vi "podControl_9066.vi"() -> ()   [LabVIEW 2016]
uses:
  <vilib>/platform/TimedLoop/XDataNode/XDataNode.xnode
  <vilib>/Platform/TimedLoop/XDataNode/nitl_modes.ctl
  <vilib>/Platform/TimedLoop/XDataNode/XDNodeRunTimeDep.lvlib
  <vilib>/Platform/TimedLoop/XDataNode/wakeup.ctl
  <vilib>/Platform/TimedLoop/XDataNode/timing_clust.ctl
  podGlobals_9066.vi
  <vilib>/Platform/TimedLoop/XDataNode/loadnilvce.vi
panel:
  out "Fatality":bool
  in  "Kill":bool
  out "Velocity":bool
  out "Acceleration":bool
  out "Battery Voltage":bool
  out "Internal Pressure":bool
  out "Internal Temperature":bool
  out "Battery Pressure":bool
  out "Battery Temperature":bool
  in  "Latch":bool
  out "Coast Time (s)":dbl
  out "Start Time (s)":dbl
  out "On Time (s)":dbl
  out "FR:":dbl
  out "BL:":dbl
  out "FL:":dbl
  out "BR:":dbl
  in  "Coast (s)":dbl
  in  "RESET":bool
  in  "Velocity (m/s)":dbl
  in  "Timeout (s)":dbl
  out "Internal Pressure (atm)":dbl(slide) scale=0.0..2.0
  out "Internal Temperature (F)":dbl(slide) scale=50.0..120.0
  out "READY":bool
  out "Flight Time (s)":dbl
  in  "START":bool
  out "Acceleration (m/s^2)":dbl(knob) scale=-30.0..30.0
  out "Position (m)":dbl
  out "Velocity (m/s)":dbl(knob) scale=0.0..300.0
  out "Latched":bool
  out "Pusher Engaged":bool
  out "Front Brake Engaged":bool
  out "Back Brake Engaged":bool
  in  "Flight Profile":T1(radio)
  out "Progress":u8(slide) caption="Profile Progress" scale=0.0..100.0
  out "Battery Pressure (atm)":dbl(slide) scale=0.0..2.0
  out "Battery Temperature (F)":dbl(slide) scale=50.0..120.0
  in  "STOP":bool
  out "Battery Voltage":dbl(knob) scale=22.0..26.0
  # "Z-Height (mm)"
  # "Custom:"
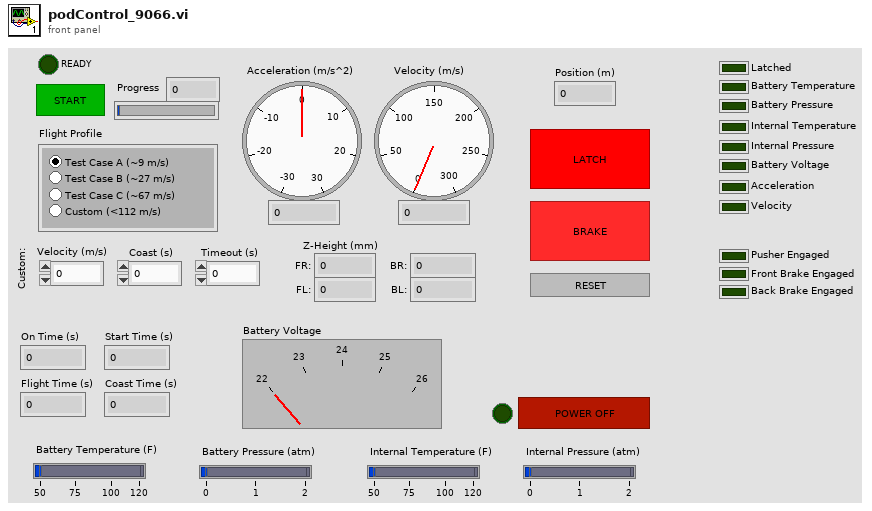
[diagram p1: front panel]
types:
  T1 = enum32{"Test Case A (~9 m/s)", "Test Case B (~27 m/s)", "Test Case C (~67 m/s)", "Custom (<112 m/s)"}
  T2 = typedef "XDNodeRunTimeDep.lvlib/timing_clust.ctl" = cluster{"Expected End [f-1]":u64, "Actual End [f-1]":u64, "Finished Late? [f-1]":bool, "Expected End [i-1]":u64, "Actual End [i-1]":u64, "Finished Late? [i-1]":bool, "Expected Start [i]":u64, "Actual Start [i]":u64, "Expected Start [f]":u64, "Actual Start [f]":u64, "Source Name":string, "Structure Name":string, "Period":i64, "Deadline":i64, "Offset":i64, "Start":i64, "Priority":i32, "Timeout":i32, "Mode":T3, "Wakeup Reason":T4, "Error":errorcluster, "Source Type":string, "Secondary Source Type":string, "Global End Time":u64, "Global Start Time":u64, "Frame Duration":u64, "Iteration Duration":u64, "Assigned CPU":i32, "I/O Scan Engine Mode":u32}
  T3 = typedef "XDNodeRunTimeDep.lvlib/nitl_modes.ctl" = enum32{"No Change", "Process missed periods, maintain original phase", "Discard missed periods, maintain original phase", "Process missed periods, ignore original phase", "Discard missed periods, ignore original phase"}
  T4 = typedef "XDNodeRunTimeDep.lvlib/wakeup.ctl" = enum32{"Normal", "Aborted", "Asynchronous wakeup", "Timing source error", "Timed loop error", "Timeout"}
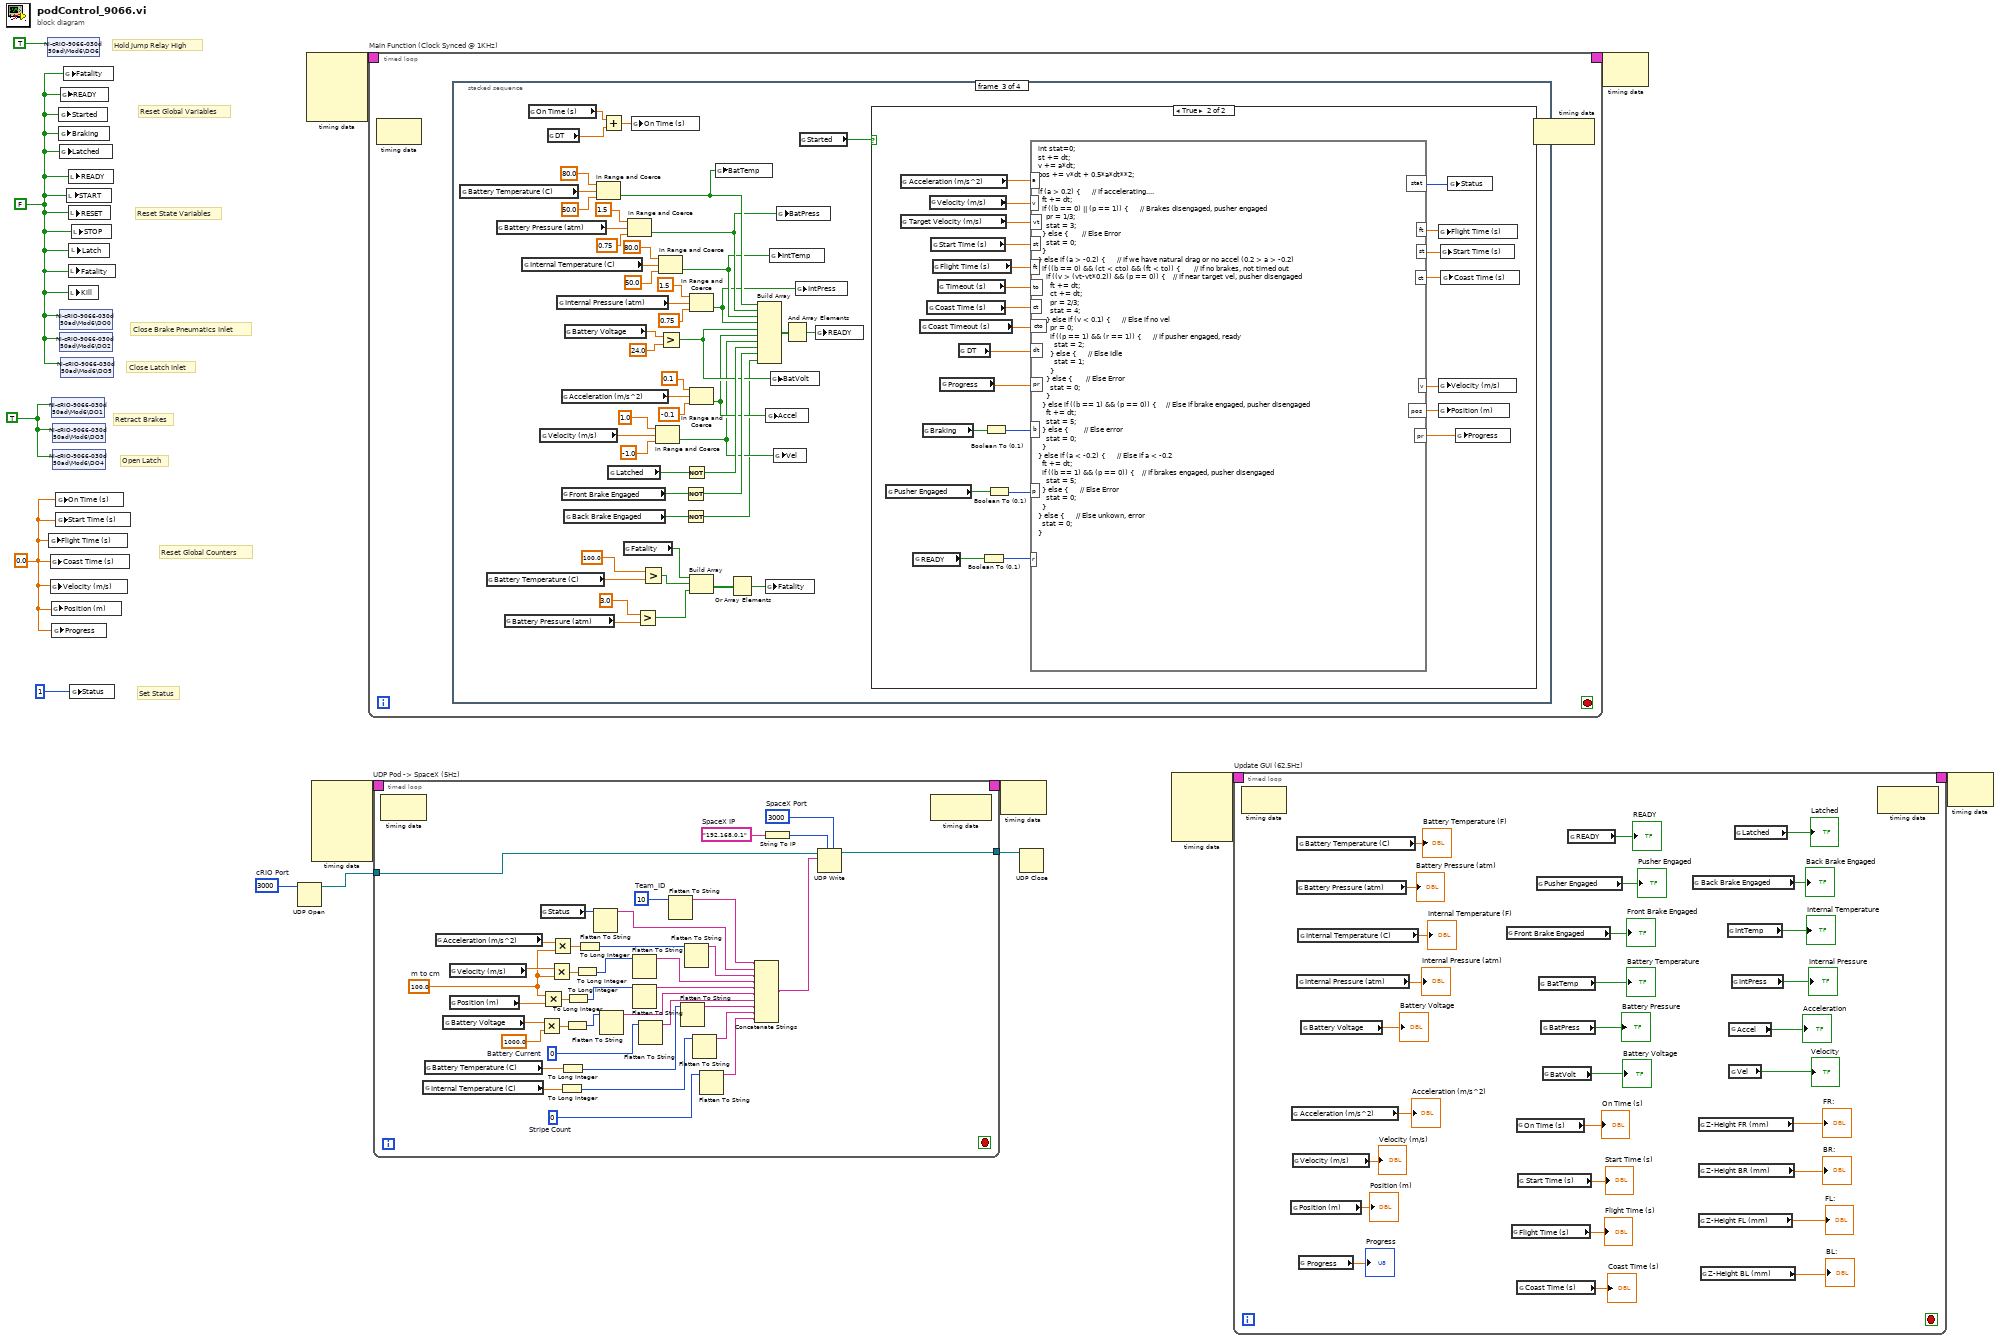
[diagram p0: block diagram]
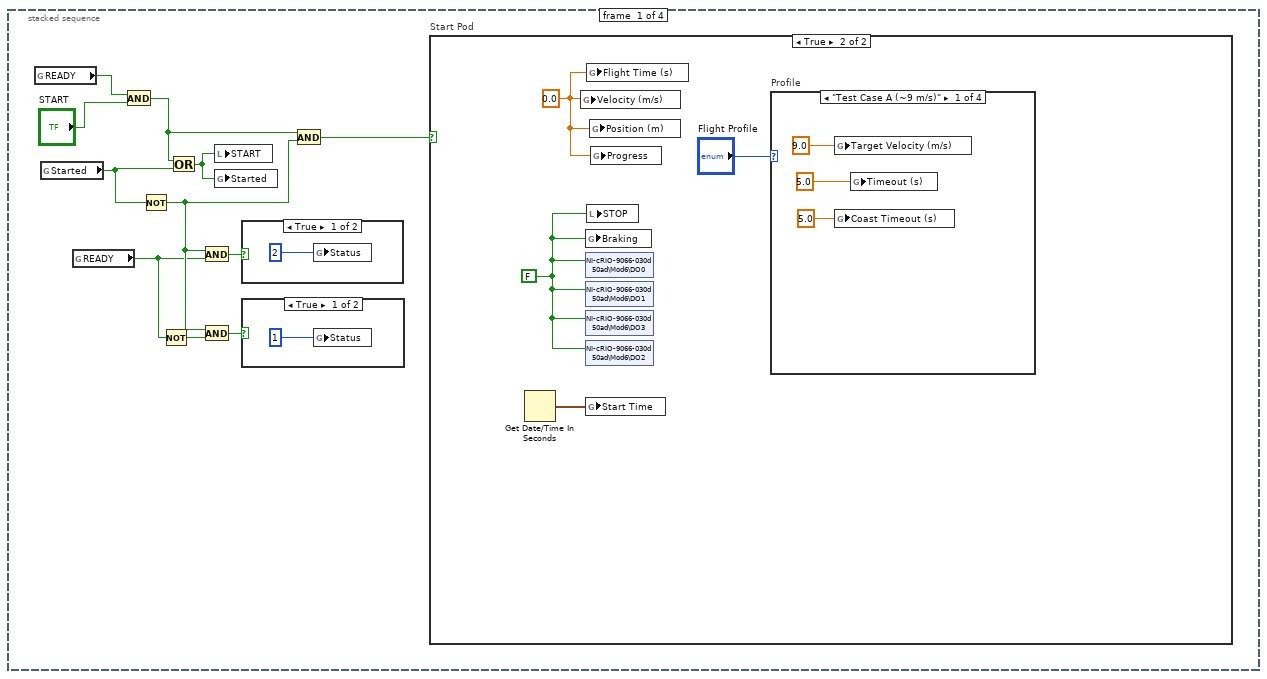
[diagram p2: hidden frame]
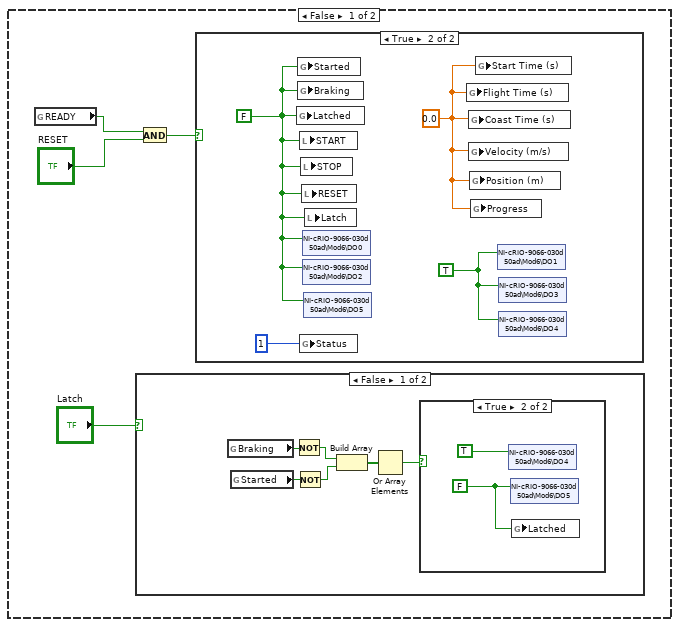
[diagram p5: hidden frame]
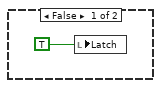
[diagram p6: hidden frame]
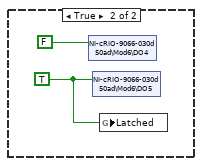
[diagram p7: hidden frame]
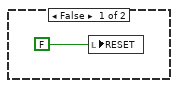
[diagram p8: hidden frame]
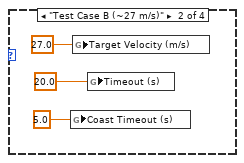
[diagram p9: hidden frame]
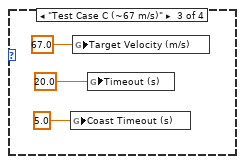
[diagram p10: hidden frame]
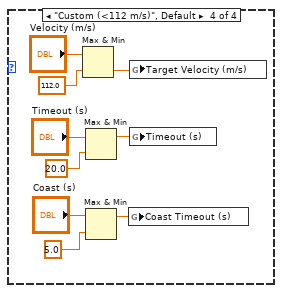
[diagram p11: hidden frame]
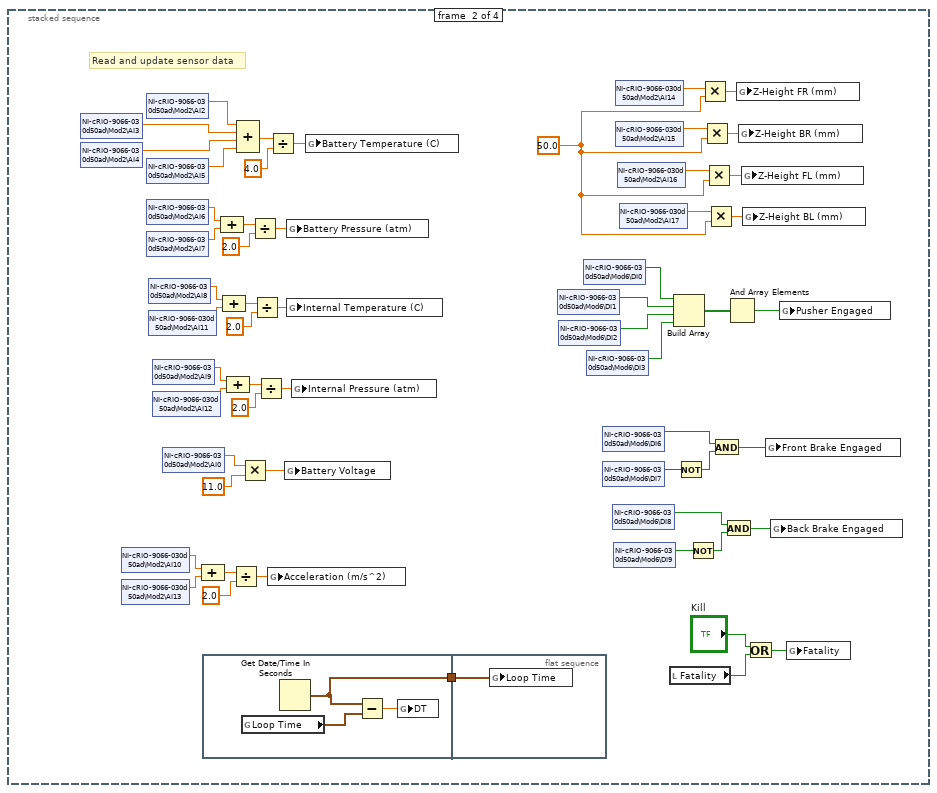
[diagram p12: hidden frame]
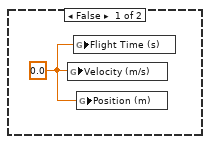
[diagram p13: hidden frame]
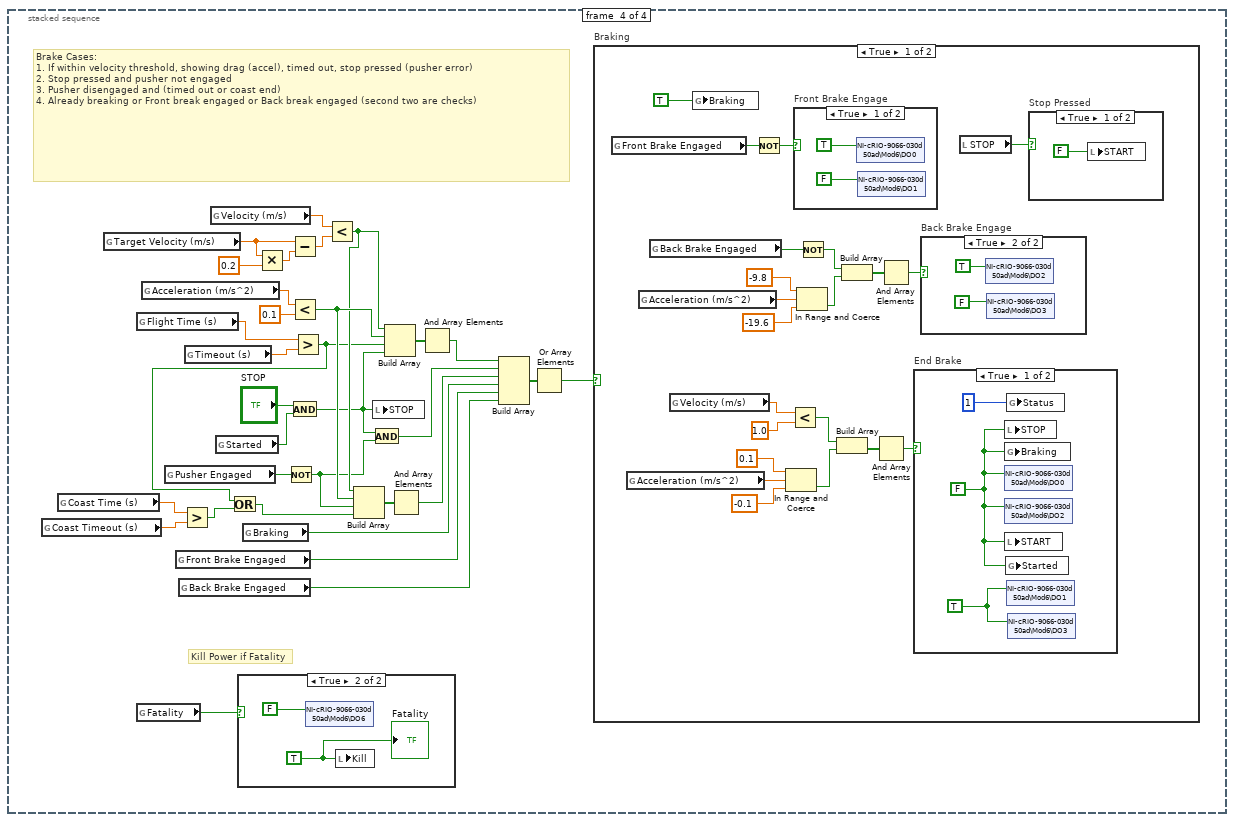
[diagram p14: hidden frame]
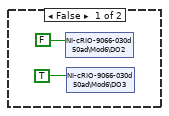
[diagram p16: hidden frame]
diagram:
  w3 = TRUE
  w10 = u32 3000  # cRIO Port
  w1 = FALSE
  w8 = 0.0
  # "Hold Jump Relay High"
  # "Close Latch Inlet"
  # "Open Latch"
  # "Set Status"
  # "Reset Global Counters"
  # "Reset Global Variables"
  # "Reset State Variables"
  # "Close Brake Pneumatics Inlet"
  # "Retract Brakes"
  n1 = shared-variable "NI-cRIO-9066-030d50ad\\Mod6\\DO6"(TRUE) -> ()  [unwired: 1 in, 1 out]
  n2 = global write "podGlobals_9066.vi" "Flight Time (s)"(w8) -> ()
  n3 = global write "podGlobals_9066.vi" "Coast Time (s)"(w8) -> ()
  n4 = global write "podGlobals_9066.vi" "Velocity (m/s)"(w8) -> ()
  n5 = global write "podGlobals_9066.vi" "Position (m)"(w8) -> ()
  n6 = shared-variable "NI-cRIO-9066-030d50ad\\Mod6\\DO1"(w3) -> ()  [unwired: 1 in, 1 out]
  n7 = global write "podGlobals_9066.vi" "Progress"(w8) -> ()
  n8 = shared-variable "NI-cRIO-9066-030d50ad\\Mod6\\DO3"(w3) -> ()  [unwired: 1 in, 1 out]
  n9 = shared-variable "NI-cRIO-9066-030d50ad\\Mod6\\DO4"(w3) -> ()  [unwired: 1 in, 1 out]
  n10 = global write "podGlobals_9066.vi" "On Time (s)"(w8) -> ()
  n11 = global write "podGlobals_9066.vi" "Start Time (s)"(w8) -> ()
  n12 = global write "podGlobals_9066.vi" "Started"(w1) -> ()
  n13 = global write "podGlobals_9066.vi" "Braking"(w1) -> ()
  n14 = global write "podGlobals_9066.vi" "Latched"(w1) -> ()
  n15 = shared-variable "NI-cRIO-9066-030d50ad\\Mod6\\DO0"(w1) -> ()  [unwired: 1 in, 1 out]
  n16 = shared-variable "NI-cRIO-9066-030d50ad\\Mod6\\DO2"(w1) -> ()  [unwired: 1 in, 1 out]
  n17 = global write "podGlobals_9066.vi" "READY"(w1) -> ()
  n18 = shared-variable "NI-cRIO-9066-030d50ad\\Mod6\\DO5"(w1) -> ()  [unwired: 1 in, 1 out]
  n19 = global write "podGlobals_9066.vi" "Fatality"(w1) -> ()
  n20 = local write "START"(w1) -> ()
  n21 = local write "READY"(w1) -> ()
  n22 = local write "RESET"(w1) -> ()
  n23 = local write "Fatality"(w1) -> ()
  n24 = local write "Kill"(w1) -> ()
  n25 = local write "Latch"(w1) -> ()
  n26 = global write "podGlobals_9066.vi" "Status"(1) -> ()
  n27 = local write "STOP"(w1) -> ()
  n28 = UDP Open(11:w10) -> (port=w5:refnum<k16>)  [unwired: 4 in, 2 out]
  n29 = node-c288() -> (w14:T2)  [unwired: 4 in]
  n30 = node-c288() -> (w12:T2)  [unwired: 5 in]
  n31 = timed-loop "Main Function (Clock Synced @ 1KHz)" {
    timing: w14 -> [_]
    timing-out: [_] -> w13
    stop <- _ stop-if-true
    n32 = node-c288() -> ()  [unwired: 1 in, 1 out]
    n33 = stacked-sequence {
      frame #0 {
        n34 = global read "podGlobals_9066.vi" "READY"() -> (w24:bool)
        n35 = global read "podGlobals_9066.vi" "Started"() -> (w25:bool)
        n36 = global read "podGlobals_9066.vi" "READY"() -> (w15:bool)
        n37 = And(x=w24, y="START") -> (x .and. y?=w21:bool)
        n38 = Not(x=w25) -> (.not. x?=w17:bool)
        n39 = Not(x=w15) -> (.not. x?=w16:bool)
        n40 = Or(x=w21, y=w25) -> (x .or. y?=w20:bool)
        n41 = And(x=w17, y=w15) -> (x .and. y?=w19:bool)
        n42 = And(x=w17, y=w16) -> (x .and. y?=w18:bool)
        n43 = local write "START"(w20) -> ()
        n44 = global write "podGlobals_9066.vi" "Started"(w20) -> ()
        n45 = case shown="True" w19 {
          frame True {
            n46 = global write "podGlobals_9066.vi" "Status"(2) -> ()
          }
          frame False {
          }
        }
        n47 = case shown="True" w18 {
          frame True {
            n48 = global write "podGlobals_9066.vi" "Status"(1) -> ()
          }
          frame False {
          }
        }
        n49 = And(x=w21, y=w17) -> (x .and. y?=w22:bool)
        n50 = case "Start Pod" shown="True" w22 {
          frame False {
            n51 = global read "podGlobals_9066.vi" "READY"() -> (w30:bool)
            n52 = case shown="False" "Latch" {
              frame False {
                n53 = global read "podGlobals_9066.vi" "Braking"() -> (w37:bool)
                n54 = global read "podGlobals_9066.vi" "Started"() -> (w36:bool)
                n55 = Not(x=w37) -> (.not. x?=w34:bool)
                n56 = Not(x=w36) -> (.not. x?=w35:bool)
                n57 = Build Array(w34, w35) -> (w33:bool[])
                n58 = Or Array Elements(Boolean array=w33) -> (logical OR=w32:bool)
                n59 = case shown="True" w32 {
                  frame False {
                    n60 = local write "Latch"(TRUE) -> ()
                  }
                  frame True {
                    w39 = FALSE
                    n61 = shared-variable "NI-cRIO-9066-030d50ad\\Mod6\\DO4"(TRUE) -> ()  [unwired: 1 in, 1 out]
                    n62 = shared-variable "NI-cRIO-9066-030d50ad\\Mod6\\DO5"(w39) -> ()  [unwired: 1 in, 1 out]
                    n63 = global write "podGlobals_9066.vi" "Latched"(w39) -> ()
                  }
                }
              }
              frame True {
                w41 = TRUE
                n64 = shared-variable "NI-cRIO-9066-030d50ad\\Mod6\\DO4"(FALSE) -> ()  [unwired: 1 in, 1 out]
                n65 = shared-variable "NI-cRIO-9066-030d50ad\\Mod6\\DO5"(w41) -> ()  [unwired: 1 in, 1 out]
                n66 = global write "podGlobals_9066.vi" "Latched"(w41) -> ()
              }
            }
            n67 = And(x=w30, y="RESET") -> (x .and. y?=w29:bool)
            n68 = case shown="True" w29 {
              frame False {
                n69 = local write "RESET"(FALSE) -> ()
              }
              frame True {
                w45 = TRUE
                w46 = 0.0
                w44 = FALSE
                n70 = global write "podGlobals_9066.vi" "Latched"(w44) -> ()
                n71 = global write "podGlobals_9066.vi" "Started"(w44) -> ()
                n72 = global write "podGlobals_9066.vi" "Braking"(w44) -> ()
                n73 = local write "START"(w44) -> ()
                n74 = global write "podGlobals_9066.vi" "Status"(1) -> ()
                n75 = local write "STOP"(w44) -> ()
                n76 = local write "RESET"(w44) -> ()
                n77 = shared-variable "NI-cRIO-9066-030d50ad\\Mod6\\DO0"(w44) -> ()  [unwired: 1 in, 1 out]
                n78 = shared-variable "NI-cRIO-9066-030d50ad\\Mod6\\DO2"(w44) -> ()  [unwired: 1 in, 1 out]
                n79 = shared-variable "NI-cRIO-9066-030d50ad\\Mod6\\DO5"(w44) -> ()  [unwired: 1 in, 1 out]
                n80 = local write "Latch"(w44) -> ()
                n81 = global write "podGlobals_9066.vi" "Flight Time (s)"(w46) -> ()
                n82 = global write "podGlobals_9066.vi" "Coast Time (s)"(w46) -> ()
                n83 = global write "podGlobals_9066.vi" "Velocity (m/s)"(w46) -> ()
                n84 = global write "podGlobals_9066.vi" "Position (m)"(w46) -> ()
                n85 = global write "podGlobals_9066.vi" "Progress"(w46) -> ()
                n86 = global write "podGlobals_9066.vi" "Start Time (s)"(w46) -> ()
                n87 = shared-variable "NI-cRIO-9066-030d50ad\\Mod6\\DO1"(w45) -> ()  [unwired: 1 in, 1 out]
                n88 = shared-variable "NI-cRIO-9066-030d50ad\\Mod6\\DO3"(w45) -> ()  [unwired: 1 in, 1 out]
                n89 = shared-variable "NI-cRIO-9066-030d50ad\\Mod6\\DO4"(w45) -> ()  [unwired: 1 in, 1 out]
              }
            }
          }
          frame True {
            w50 = FALSE
            w49 = 0.0
            n90 = Get Date/Time In Seconds() -> (seconds since 1Jan1904=w48:timestamp)
            n91 = global write "podGlobals_9066.vi" "Velocity (m/s)"(w49) -> ()
            n92 = global write "podGlobals_9066.vi" "Braking"(w50) -> ()
            n93 = shared-variable "NI-cRIO-9066-030d50ad\\Mod6\\DO0"(w50) -> ()  [unwired: 1 in, 1 out]
            n94 = shared-variable "NI-cRIO-9066-030d50ad\\Mod6\\DO1"(w50) -> ()  [unwired: 1 in, 1 out]
            n95 = shared-variable "NI-cRIO-9066-030d50ad\\Mod6\\DO3"(w50) -> ()  [unwired: 1 in, 1 out]
            n96 = shared-variable "NI-cRIO-9066-030d50ad\\Mod6\\DO2"(w50) -> ()  [unwired: 1 in, 1 out]
            n97 = global write "podGlobals_9066.vi" "Start Time"(w48) -> ()
            n98 = global write "podGlobals_9066.vi" "Flight Time (s)"(w49) -> ()
            n99 = local write "STOP"(w50) -> ()
            n100 = global write "podGlobals_9066.vi" "Position (m)"(w49) -> ()
            n101 = global write "podGlobals_9066.vi" "Progress"(w49) -> ()
            n102 = case "Profile" shown="\"Test Case A (~9 m/s)\"" "Flight Profile" {
              frame "Test Case A (~9 m/s)" {
                n103 = global write "podGlobals_9066.vi" "Target Velocity (m/s)"(9.0) -> ()
                n104 = global write "podGlobals_9066.vi" "Coast Timeout (s)"(5.0) -> ()
                n105 = global write "podGlobals_9066.vi" "Timeout (s)"(5.0) -> ()
              }
              frame "Test Case B (~27 m/s)" {
                n106 = global write "podGlobals_9066.vi" "Coast Timeout (s)"(5.0) -> ()
                n107 = global write "podGlobals_9066.vi" "Target Velocity (m/s)"(27.0) -> ()
                n108 = global write "podGlobals_9066.vi" "Timeout (s)"(20.0) -> ()
              }
              frame "Test Case C (~67 m/s)" {
                n109 = global write "podGlobals_9066.vi" "Coast Timeout (s)"(5.0) -> ()
                n110 = global write "podGlobals_9066.vi" "Target Velocity (m/s)"(67.0) -> ()
                n111 = global write "podGlobals_9066.vi" "Timeout (s)"(20.0) -> ()
              }
              frame "Custom (<112 m/s)", Default {
                n112 = Max & Min(x="Velocity (m/s)", y=112.0) -> (min(x,y)=w63:dbl)  [unwired: 1 out]
                n113 = Max & Min(x="Timeout (s)", y=20.0) -> (max(x,y)=w69:dbl)  [unwired: 1 out]
                n114 = Max & Min(x="Coast (s)", y=5.0) -> (max(x,y)=w66:dbl)  [unwired: 1 out]
                n115 = global write "podGlobals_9066.vi" "Coast Timeout (s)"(w66) -> ()
                n116 = global write "podGlobals_9066.vi" "Target Velocity (m/s)"(w63) -> ()
                n117 = global write "podGlobals_9066.vi" "Timeout (s)"(w69) -> ()
              }
            }
          }
        }
      }
      frame #1 {
        w82 = 50.0
        # "Read and update sensor data"
        n118 = shared-variable "NI-cRIO-9066-030d50ad\\Mod2\\AI3"() -> (w109:dbl)  [unwired: 1 in, 1 out]
        n119 = shared-variable "NI-cRIO-9066-030d50ad\\Mod2\\AI4"() -> (w110:dbl)  [unwired: 1 in, 1 out]
        n120 = shared-variable "NI-cRIO-9066-030d50ad\\Mod2\\AI10"() -> (w119:dbl)  [unwired: 1 in, 1 out]
        n121 = shared-variable "NI-cRIO-9066-030d50ad\\Mod2\\AI13"() -> (w120:dbl)  [unwired: 1 in, 1 out]
        n122 = shared-variable "NI-cRIO-9066-030d50ad\\Mod2\\AI2"() -> (w97:dbl)  [unwired: 1 in, 1 out]
        n123 = shared-variable "NI-cRIO-9066-030d50ad\\Mod2\\AI5"() -> (w111:dbl)  [unwired: 1 in, 1 out]
        n124 = shared-variable "NI-cRIO-9066-030d50ad\\Mod2\\AI6"() -> (w114:dbl)  [unwired: 1 in, 1 out]
        n125 = shared-variable "NI-cRIO-9066-030d50ad\\Mod2\\AI7"() -> (w115:dbl)  [unwired: 1 in, 1 out]
        n126 = shared-variable "NI-cRIO-9066-030d50ad\\Mod2\\AI8"() -> (w98:dbl)  [unwired: 1 in, 1 out]
        n127 = shared-variable "NI-cRIO-9066-030d50ad\\Mod2\\AI11"() -> (w99:dbl)  [unwired: 1 in, 1 out]
        n128 = shared-variable "NI-cRIO-9066-030d50ad\\Mod2\\AI9"() -> (w103:dbl)  [unwired: 1 in, 1 out]
        n129 = shared-variable "NI-cRIO-9066-030d50ad\\Mod2\\AI12"() -> (w104:dbl)  [unwired: 1 in, 1 out]
        n130 = shared-variable "NI-cRIO-9066-030d50ad\\Mod2\\AI0"() -> (w124:dbl)  [unwired: 1 in, 1 out]
        n131 = Compound Arithmetic op=ADD(w119, w120) -> (w121:dbl)
        n132 = flat-sequence {
          tunnel: [w127] -> w81
          tunnel: w81 -> [w130]
          frame #0 {
            n133 = global read "podGlobals_9066.vi" "Loop Time"() -> (w129:timestamp)
            n134 = Get Date/Time In Seconds() -> (seconds since 1Jan1904=w127:timestamp)
            n135 = Subtract(x=w127, y=w129) -> (x-y=w128:dbl)
            n136 = global write "podGlobals_9066.vi" "DT"(w128) -> ()
          }
          frame #1 {
            n137 = global write "podGlobals_9066.vi" "Loop Time"(w130) -> ()
          }
        }
        n138 = Compound Arithmetic op=ADD(w114, w115) -> (w116:dbl)
        n139 = Compound Arithmetic op=ADD(w98, w99) -> (w100:dbl)
        n140 = Compound Arithmetic op=ADD(w103, w104) -> (w105:dbl)
        n141 = Divide(x=w121, y=2.0) -> (x/y=w123:dbl)
        n142 = Compound Arithmetic op=ADD(w97, w109, w110, w111) -> (w108:dbl)
        n143 = Multiply(x=w124, y=11.0) -> (x*y=w126:dbl)
        n144 = Divide(x=w116, y=2.0) -> (x/y=w118:dbl)
        n145 = Divide(x=w100, y=2.0) -> (x/y=w102:dbl)
        n146 = Divide(x=w105, y=2.0) -> (x/y=w107:dbl)
        n147 = Divide(x=w108, y=4.0) -> (x/y=w113:dbl)
        n148 = global write "podGlobals_9066.vi" "Acceleration (m/s^2)"(w123) -> ()
        n149 = global write "podGlobals_9066.vi" "Battery Voltage"(w126) -> ()
        n150 = global write "podGlobals_9066.vi" "Battery Pressure (atm)"(w118) -> ()
        n151 = global write "podGlobals_9066.vi" "Internal Temperature (C)"(w102) -> ()
        n152 = global write "podGlobals_9066.vi" "Internal Pressure (atm)"(w107) -> ()
        n153 = global write "podGlobals_9066.vi" "Battery Temperature (C)"(w113) -> ()
        n154 = shared-variable "NI-cRIO-9066-030d50ad\\Mod6\\DI1"() -> (w95:bool)  [unwired: 1 in, 1 out]
        n155 = shared-variable "NI-cRIO-9066-030d50ad\\Mod6\\DI2"() -> (w94:bool)  [unwired: 1 in, 1 out]
        n156 = shared-variable "NI-cRIO-9066-030d50ad\\Mod6\\DI0"() -> (w96:bool)  [unwired: 1 in, 1 out]
        n157 = shared-variable "NI-cRIO-9066-030d50ad\\Mod6\\DI3"() -> (w93:bool)  [unwired: 1 in, 1 out]
        n158 = shared-variable "NI-cRIO-9066-030d50ad\\Mod6\\DI6"() -> (w78:bool)  [unwired: 1 in, 1 out]
        n159 = shared-variable "NI-cRIO-9066-030d50ad\\Mod6\\DI7"() -> (w77:bool)  [unwired: 1 in, 1 out]
        n160 = shared-variable "NI-cRIO-9066-030d50ad\\Mod6\\DI8"() -> (w75:bool)  [unwired: 1 in, 1 out]
        n161 = shared-variable "NI-cRIO-9066-030d50ad\\Mod6\\DI9"() -> (w74:bool)  [unwired: 1 in, 1 out]
        n162 = shared-variable "NI-cRIO-9066-030d50ad\\Mod2\\AI14"() -> (w89:dbl)  [unwired: 1 in, 1 out]
        n163 = shared-variable "NI-cRIO-9066-030d50ad\\Mod2\\AI15"() -> (w85:dbl)  [unwired: 1 in, 1 out]
        n164 = shared-variable "NI-cRIO-9066-030d50ad\\Mod2\\AI16"() -> (w84:dbl)  [unwired: 1 in, 1 out]
        n165 = shared-variable "NI-cRIO-9066-030d50ad\\Mod2\\AI17"() -> (w83:dbl)  [unwired: 1 in, 1 out]
        n166 = local read "Fatality"() -> (w70:bool)
        n167 = Build Array(w96, w95, w94, w93) -> (w92:bool[])
        n168 = Not(x=w77) -> (.not. x?=w80:bool)
        n169 = Not(x=w74) -> (.not. x?=w79:bool)
        n170 = Multiply(x=w89, y=w82) -> (x*y=w90:dbl)
        n171 = Multiply(x=w85, y=w82) -> (x*y=w88:dbl)
        n172 = Multiply(x=w84, y=w82) -> (x*y=w87:dbl)
        n173 = Multiply(x=w83, y=w82) -> (x*y=w86:dbl)
        n174 = And(x=w78, y=w80) -> (x .and. y?=w76:bool)
        n175 = And(x=w75, y=w79) -> (x .and. y?=w73:bool)
        n176 = And Array Elements(Boolean array=w92) -> (logical AND=w91:bool)
        n177 = global write "podGlobals_9066.vi" "Z-Height FR (mm)"(w90) -> ()
        n178 = global write "podGlobals_9066.vi" "Z-Height BR (mm)"(w88) -> ()
        n179 = global write "podGlobals_9066.vi" "Z-Height FL (mm)"(w87) -> ()
        n180 = global write "podGlobals_9066.vi" "Z-Height BL (mm)"(w86) -> ()
        n181 = Or(x="Kill", y=w70) -> (x .or. y?=w72:bool)
        n182 = global write "podGlobals_9066.vi" "Front Brake Engaged"(w76) -> ()
        n183 = global write "podGlobals_9066.vi" "Back Brake Engaged"(w73) -> ()
        n184 = global write "podGlobals_9066.vi" "Pusher Engaged"(w91) -> ()
        n185 = global write "podGlobals_9066.vi" "Fatality"(w72) -> ()
      }
      frame #2 {
        n186 = global read "podGlobals_9066.vi" "Battery Temperature (C)"() -> (w167:dbl)
        n187 = global read "podGlobals_9066.vi" "Battery Temperature (C)"() -> (w137:dbl)
        n188 = global read "podGlobals_9066.vi" "Battery Pressure (atm)"() -> (w170:dbl)
        n189 = global read "podGlobals_9066.vi" "Battery Pressure (atm)"() -> (w139:dbl)
        n190 = global read "podGlobals_9066.vi" "Internal Temperature (C)"() -> (w161:dbl)
        n191 = global read "podGlobals_9066.vi" "On Time (s)"() -> (w151:dbl)
        n192 = global read "podGlobals_9066.vi" "Velocity (m/s)"() -> (w155:dbl)
        n193 = global read "podGlobals_9066.vi" "DT"() -> (w149:dbl)
        n194 = global read "podGlobals_9066.vi" "Internal Pressure (atm)"() -> (w164:dbl)
        n195 = global read "podGlobals_9066.vi" "Acceleration (m/s^2)"() -> (w173:dbl)
        n196 = global read "podGlobals_9066.vi" "Front Brake Engaged"() -> (w158:bool)
        n197 = global read "podGlobals_9066.vi" "Back Brake Engaged"() -> (w159:bool)
        n198 = global read "podGlobals_9066.vi" "Battery Voltage"() -> (w176:dbl)
        n199 = In Range and Coerce(upper limit=80.0, x=w167, lower limit=50.0) -> (In Range?=w147:bool)  [unwired: 1 out]
        n200 = Add(x=w151, y=w149) -> (x+y=w150:dbl)
        n201 = global read "podGlobals_9066.vi" "Latched"() -> (w153:bool)
        n202 = global read "podGlobals_9066.vi" "Fatality"() -> (w134:bool)
        n203 = In Range and Coerce(upper limit=1.5, x=w170, lower limit=0.75) -> (In Range?=w146:bool)  [unwired: 1 out]
        n204 = global write "podGlobals_9066.vi" "On Time (s)"(w150) -> ()
        n205 = Greater?(x=3.0, y=w139) -> (0:w131:bool)
        n206 = Greater?(x=100.0, y=w137) -> (0:w132:bool)
        n207 = In Range and Coerce(upper limit=1.0, x=w155, lower limit=-1.0) -> (In Range?=w141:bool)  [unwired: 1 out]
        n208 = In Range and Coerce(upper limit=80.0, x=w161, lower limit=50.0) -> (In Range?=w145:bool)  [unwired: 1 out]
        n209 = Greater?(x=w176, y=24.0) -> (0:w143:bool)
        n210 = Not(x=w158) -> (.not. x?=w154:bool)
        n211 = Not(x=w159) -> (.not. x?=w135:bool)
        n212 = Not(x=w153) -> (.not. x?=w152:bool)
        n213 = In Range and Coerce(upper limit=1.5, x=w164, lower limit=0.75) -> (In Range?=w144:bool)  [unwired: 1 out]
        n214 = In Range and Coerce(upper limit=0.1, x=w173, lower limit=-0.1) -> (In Range?=w142:bool)  [unwired: 1 out]
        n215 = Build Array(w134, w132, w131) -> (w136:bool[])
        n216 = global write "podGlobals_9066.vi" "BatTemp"(w147) -> ()
        n217 = Or Array Elements(Boolean array=w136) -> (logical OR=w133:bool)
        n218 = Build Array(w147, w146, w145, w144, w143, w142, w141, w152, w154, w135) -> (w160:bool[])
        n219 = global write "podGlobals_9066.vi" "Fatality"(w133) -> ()
        n220 = global write "podGlobals_9066.vi" "Accel"(w142) -> ()
        n221 = global write "podGlobals_9066.vi" "IntTemp"(w145) -> ()
        n222 = global write "podGlobals_9066.vi" "BatVolt"(w143) -> ()
        n223 = global write "podGlobals_9066.vi" "Vel"(w141) -> ()
        n224 = global write "podGlobals_9066.vi" "BatPress"(w146) -> ()
        n225 = And Array Elements(Boolean array=w160) -> (logical AND=w148:bool)
        n226 = global write "podGlobals_9066.vi" "IntPress"(w144) -> ()
        n227 = global read "podGlobals_9066.vi" "Started"() -> (w178:bool)
        n228 = global write "podGlobals_9066.vi" "READY"(w148) -> ()
        n229 = case shown="True" w178 {
          frame False {
            w179 = 0.0
            n230 = global write "podGlobals_9066.vi" "Velocity (m/s)"(w179) -> ()
            n231 = global write "podGlobals_9066.vi" "Flight Time (s)"(w179) -> ()
            n232 = global write "podGlobals_9066.vi" "Position (m)"(w179) -> ()
          }
          frame True {
            n233 = global read "podGlobals_9066.vi" "Pusher Engaged"() -> (w182:bool)
            n234 = global read "podGlobals_9066.vi" "Acceleration (m/s^2)"() -> (w202:dbl)
            n235 = global read "podGlobals_9066.vi" "Target Velocity (m/s)"() -> (w200:dbl)
            n236 = global read "podGlobals_9066.vi" "READY"() -> (w181:bool)
            n237 = global read "podGlobals_9066.vi" "Coast Timeout (s)"() -> (w187:dbl)
            n238 = global read "podGlobals_9066.vi" "Braking"() -> (w185:bool)
            n239 = global read "podGlobals_9066.vi" "Coast Time (s)"() -> (w195:dbl)
            n240 = global read "podGlobals_9066.vi" "Velocity (m/s)"() -> (w201:dbl)
            n241 = global read "podGlobals_9066.vi" "Start Time (s)"() -> (w189:dbl)
            n242 = global read "podGlobals_9066.vi" "Flight Time (s)"() -> (w199:dbl)
            n243 = global read "podGlobals_9066.vi" "Timeout (s)"() -> (w198:dbl)
            n244 = global read "podGlobals_9066.vi" "Progress"() -> (w191:dbl)
            n245 = global read "podGlobals_9066.vi" "DT"() -> (w186:dbl)
            n246 = Boolean To (0,1)(Boolean=w181) -> (0, 1=w180:i16)
            n247 = Boolean To (0,1)(Boolean=w185) -> (0, 1=w184:i16)
            n248 = Boolean To (0,1)(Boolean=w182) -> (0, 1=w183:i16)
            n249 = formula code="int stat=0;\nst += dt;\nv += a*dt;\npos += v*dt + 0.5*a*dt**2;\n\nif (a > 0.2) {      // If accelerating....\n  ft += dt;\n  if ((b == 0) || (p == 1)) {      // Brakes disengaged, pusher engaged\n    pr = 1/3;\n    stat = 3;\n  } else {       // Else Error\n    stat = 0;\n  }\n} else if (a > -0.2) {      // If we have natural drag or no accel (0.2 > a > -0.2)\n  if ((b == 0) && (ct < cto) && (ft < to)) {       // If no brakes, not timed out\n    if ((v > (vt-vt*0.2)) && (p == 0)) {    // If near target vel, pusher disengaged\n      ft += dt;\n      ct += dt;\n      pr = 2/3;\n      stat = 4;\n    } else if (v < 0.1) {      // Else if no vel\n      pr = 0;\n      if ((p == 1) && (r == 1)) {      // If pusher engaged, ready\n        stat = 2;\n      } else {      // Else Idle\n        stat = 1;\n      }\n    } else {       // Else Error\n      stat = 0;\n    }\n  } else if ((b == 1) && (p == 0)) {     // Else if brake engaged, pusher disengaged\n    ft += dt;\n    stat = 5;\n  } else {        // Else error\n    stat = 0;\n  }\n} else if (a < -0.2) {      // Else if a < -0.2\n  ft += dt;\n  if ((b == 1) && (p == 0)) {    // If brakes engaged, pusher disengaged\n    stat = 5;\n  } else {      // Else Error\n    stat = 0;\n  }\n} else {      // Else unkown, error\n  stat = 0;\n}"("a"=w202, "v"=w201, "vt"=w200, "ft"=w199, "to"=w198, "b"=w184, "p"=w183, "ct"=w195, "r"=w180, "pr"=w191, "st"=w189, "cto"=w187, "dt"=w186) -> ("stat"=w197:i32, "ct"=w196:dbl, "ft"=w192:dbl, "v"=w193:dbl, "pos"=w194:dbl, "pr"=w190:dbl, "st"=w188:dbl)
            n250 = global write "podGlobals_9066.vi" "Flight Time (s)"(w192) -> ()
            n251 = global write "podGlobals_9066.vi" "Velocity (m/s)"(w193) -> ()
            n252 = global write "podGlobals_9066.vi" "Position (m)"(w194) -> ()
            n253 = global write "podGlobals_9066.vi" "Start Time (s)"(w188) -> ()
            n254 = global write "podGlobals_9066.vi" "Coast Time (s)"(w196) -> ()
            n255 = global write "podGlobals_9066.vi" "Status"(w197) -> ()
            n256 = global write "podGlobals_9066.vi" "Progress"(w190) -> ()
          }
        }
      }
      frame #3 {
        # "Kill Power if Fatality"
        # "Brake Cases:\n1. If within velocity threshold, showing drag (accel), timed out, stop pressed (pusher error)\n2. Stop pressed and pusher not engaged\n3. Pusher disengaged and (timed out or coast end)\n4. Already breaking or Front break engaged or Back break engaged (second two are checks)"
        n257 = global read "podGlobals_9066.vi" "Coast Timeout (s)"() -> (w208:dbl)
        n258 = global read "podGlobals_9066.vi" "Coast Time (s)"() -> (w209:dbl)
        n259 = global read "podGlobals_9066.vi" "Target Velocity (m/s)"() -> (w228:dbl)
        n260 = global read "podGlobals_9066.vi" "Flight Time (s)"() -> (w233:dbl)
        n261 = global read "podGlobals_9066.vi" "Fatality"() -> (w203:bool)
        n262 = global read "podGlobals_9066.vi" "Acceleration (m/s^2)"() -> (w231:dbl)
        n263 = global read "podGlobals_9066.vi" "Pusher Engaged"() -> (w234:bool)
        n264 = global read "podGlobals_9066.vi" "Front Brake Engaged"() -> (w220:bool)
        n265 = global read "podGlobals_9066.vi" "Back Brake Engaged"() -> (w221:bool)
        n266 = Greater?(x=w209, y=w208) -> (0:w205:bool)
        n267 = global read "podGlobals_9066.vi" "Timeout (s)"() -> (w226:dbl)
        n268 = global read "podGlobals_9066.vi" "Velocity (m/s)"() -> (w224:dbl)
        n269 = global read "podGlobals_9066.vi" "Started"() -> (w211:bool)
        n270 = case shown="True" w203 {
          frame False {
          }
          frame True {
            w235 = TRUE
            n271 = shared-variable "NI-cRIO-9066-030d50ad\\Mod6\\DO6"(FALSE) -> ()  [unwired: 1 in, 1 out]
            n272 = local write "Kill"(w235) -> ()
            "Fatality" <- w235
          }
        }
        n273 = global read "podGlobals_9066.vi" "Braking"() -> (w219:bool)
        n274 = Multiply(x=w228, y=0.2) -> (x*y=w229:dbl)
        n275 = Not(x=w234) -> (.not. x?=w207:bool)
        n276 = Subtract(x=w228, y=w229) -> (x-y=w225:dbl)
        n277 = Less?(x=w231, y=0.1) -> (x < y?=w216:bool)
        n278 = And(x="STOP", y=w211) -> (x .and. y?=w210:bool)
        n279 = Greater?(x=w233, y=w226) -> (0:w204:bool)
        n280 = Or(x=w204, y=w205) -> (x .or. y?=w206:bool)
        n281 = Less?(x=w224, y=w225) -> (x < y?=w215:bool)
        n282 = Build Array(w215, w216, w207, w206) -> (w218:bool[])
        n283 = And(x=w210, y=w207) -> (x .and. y?=w223:bool)
        n284 = local write "STOP"(w210) -> ()
        n285 = Build Array(w215, w216, w204, w210) -> (w232:bool[])
        n286 = And Array Elements(Boolean array=w218) -> (logical AND=w217:bool)
        n287 = And Array Elements(Boolean array=w232) -> (logical AND=w213:bool)
        n288 = Build Array(w213, w223, w217, w219, w220, w221) -> (w222:bool[])
        n289 = Or Array Elements(Boolean array=w222) -> (logical OR=w214:bool)
        n290 = case "Braking" shown="True" w214 {
          frame True {
            n291 = global read "podGlobals_9066.vi" "Front Brake Engaged"() -> (w246:bool)
            n292 = global read "podGlobals_9066.vi" "Acceleration (m/s^2)"() -> (w255:dbl)
            n293 = global read "podGlobals_9066.vi" "Acceleration (m/s^2)"() -> (w238:dbl)
            n294 = global read "podGlobals_9066.vi" "Back Brake Engaged"() -> (w244:bool)
            n295 = global read "podGlobals_9066.vi" "Velocity (m/s)"() -> (w257:dbl)
            n296 = global write "podGlobals_9066.vi" "Braking"(TRUE) -> ()
            n297 = Not(x=w246) -> (.not. x?=w245:bool)
            n298 = In Range and Coerce(upper limit=0.1, x=w255, lower limit=-0.1) -> (In Range?=w249:bool)  [unwired: 1 out]
            n299 = Less?(x=w257, y=1.0) -> (x < y?=w250:bool)
            n300 = case "Front Brake Engage" shown="True" w245 {
              frame True {
                n301 = shared-variable "NI-cRIO-9066-030d50ad\\Mod6\\DO0"(TRUE) -> ()  [unwired: 1 in, 1 out]
                n302 = shared-variable "NI-cRIO-9066-030d50ad\\Mod6\\DO1"(FALSE) -> ()  [unwired: 1 in, 1 out]
              }
              frame False {
              }
            }
            n303 = In Range and Coerce(upper limit=-9.8, x=w238, lower limit=-19.6) -> (In Range?=w243:bool)  [unwired: 1 out]
            n304 = Not(x=w244) -> (.not. x?=w239:bool)
            n305 = Build Array(w250, w249) -> (w251:bool[])
            n306 = Build Array(w239, w243) -> (w242:bool[])
            n307 = And Array Elements(Boolean array=w251) -> (logical AND=w252:bool)
            n308 = And Array Elements(Boolean array=w242) -> (logical AND=w241:bool)
            n309 = case "End Brake" shown="True" w252 {
              frame True {
                w265 = TRUE
                w267 = FALSE
                n310 = local write "STOP"(w267) -> ()
                n311 = global write "podGlobals_9066.vi" "Braking"(w267) -> ()
                n312 = shared-variable "NI-cRIO-9066-030d50ad\\Mod6\\DO0"(w267) -> ()  [unwired: 1 in, 1 out]
                n313 = shared-variable "NI-cRIO-9066-030d50ad\\Mod6\\DO2"(w267) -> ()  [unwired: 1 in, 1 out]
                n314 = local write "START"(w267) -> ()
                n315 = global write "podGlobals_9066.vi" "Started"(w267) -> ()
                n316 = global write "podGlobals_9066.vi" "Status"(1) -> ()
                n317 = shared-variable "NI-cRIO-9066-030d50ad\\Mod6\\DO1"(w265) -> ()  [unwired: 1 in, 1 out]
                n318 = shared-variable "NI-cRIO-9066-030d50ad\\Mod6\\DO3"(w265) -> ()  [unwired: 1 in, 1 out]
              }
              frame False {
              }
            }
            n319 = case "Back Brake Engage" shown="True" w241 {
              frame False {
                n320 = shared-variable "NI-cRIO-9066-030d50ad\\Mod6\\DO2"(FALSE) -> ()  [unwired: 1 in, 1 out]
                n321 = shared-variable "NI-cRIO-9066-030d50ad\\Mod6\\DO3"(TRUE) -> ()  [unwired: 1 in, 1 out]
              }
              frame True {
                n322 = shared-variable "NI-cRIO-9066-030d50ad\\Mod6\\DO2"(TRUE) -> ()  [unwired: 1 in, 1 out]
                n323 = shared-variable "NI-cRIO-9066-030d50ad\\Mod6\\DO3"(FALSE) -> ()  [unwired: 1 in, 1 out]
              }
            }
            n324 = local read "STOP"() -> (w247:bool)
            n325 = case "Stop Pressed" shown="True" w247 {
              frame True {
                n326 = local write "START"(FALSE) -> ()
              }
              frame False {
              }
            }
          }
          frame False {
          }
        }
      }
    }
    n327 = node-c288() -> ()  [unwired: 1 in, 1 out]
  }
  n328 = timed-loop "UDP Pod -> SpaceX (5Hz)" {
    timing: w12 -> [_]
    timing-out: [_] -> w11
    tunnel: w5 -> [w271]
    tunnel: [w270] -> w4
    stop <- _ stop-if-true
    w272 = u32 0  # Stripe Count
    w278 = 0  # Battery Current
    w304 = 100.0  # m to cm
    w290 = u8 10  # Team_ID
    w292 = u16 3000  # SpaceX Port
    w295 = "192.168.0.1"  # SpaceX IP
    n329 = node-c288() -> ()  [unwired: 1 in, 1 out]
    n330 = global read "podGlobals_9066.vi" "Internal Temperature (C)"() -> (w296:dbl)
    n331 = global read "podGlobals_9066.vi" "Battery Temperature (C)"() -> (w297:dbl)
    n332 = global read "podGlobals_9066.vi" "Acceleration (m/s^2)"() -> (w307:dbl)
    n333 = global read "podGlobals_9066.vi" "Battery Voltage"() -> (w298:dbl)
    n334 = global read "podGlobals_9066.vi" "Velocity (m/s)"() -> (w306:dbl)
    n335 = global read "podGlobals_9066.vi" "Position (m)"() -> (w305:dbl)
    n336 = Multiply(x=w298, y=1000.0) -> (x*y=w300:dbl)
    n337 = global read "podGlobals_9066.vi" "Status"() -> (w288:u8)
    n338 = Multiply(x=w304, y=w305) -> (x*y=w301:dbl)
    n339 = Multiply(x=w306, y=w304) -> (x*y=w302:dbl)
    n340 = Multiply(x=w307, y=w304) -> (x*y=w303:dbl)
    n341 = To Long Integer(number=w296) -> (32bit integer=w274:i32)
    n342 = To Long Integer(number=w297) -> (32bit integer=w276:i32)
    n343 = To Long Integer(number=w300) -> (32bit integer=w280:i32)
    n344 = To Long Integer(number=w301) -> (32bit integer=w282:i32)
    n345 = To Long Integer(number=w302) -> (32bit integer=w284:i32)
    n346 = To Long Integer(number=w303) -> (32bit integer=w287:i32)
    n347 = Flatten To String(anything=w288) -> (data string=w289:string)  [unwired: 3 in, 2 out]
    n348 = Flatten To String(anything=w280) -> (data string=w281:string)  [unwired: 3 in, 2 out]
    n349 = Flatten To String(anything=w284) -> (data string=w285:string)  [unwired: 3 in, 2 out]
    n350 = Flatten To String(anything=w282) -> (data string=w283:string)  [unwired: 3 in, 2 out]
    n351 = Flatten To String(anything=w278) -> (data string=w279:string)  [unwired: 3 in, 2 out]
    n352 = Flatten To String(anything=w290) -> (data string=w291:string)  [unwired: 3 in, 2 out]
    n353 = Flatten To String(anything=w276) -> (data string=w277:string)  [unwired: 3 in, 2 out]
    n354 = Flatten To String(anything=w287) -> (data string=w286:string)  [unwired: 3 in, 2 out]
    n355 = Flatten To String(anything=w274) -> (data string=w275:string)  [unwired: 3 in, 2 out]
    n356 = Flatten To String(anything=w272) -> (data string=w273:string)  [unwired: 3 in, 2 out]
    n357 = Concatenate Strings(w291, w289, w286, w285, w283, w281, w279, w277, w275, w273) -> (w294:string)
    n358 = String To IP(1:w295) -> (0:w293:u32)
    n359 = UDP Write(address=w293, port or service name=w292, connection ID=w271, data in=w294) -> (3:w270:refnum<k16>)  [unwired: 2 in, 1 out]
    n360 = node-c288() -> ()  [unwired: 1 in, 1 out]
  }
  n361 = node-c288(w11) -> ()  [unwired: 1 out]
  n362 = UDP Close(connection ID=w4) -> ()  [unwired: 1 in, 2 out]
  n363 = node-c288() -> (w7:T2)  [unwired: 4 in]
  n364 = timed-loop "Update GUI (62.5Hz)" {
    timing: w7 -> [_]
    timing-out: [_] -> w6
    stop <- _ stop-if-true
    n365 = node-c288() -> ()  [unwired: 1 in, 1 out]
    n366 = global read "podGlobals_9066.vi" "Position (m)"() -> (→"Position (m)":dbl)
    n367 = global read "podGlobals_9066.vi" "Acceleration (m/s^2)"() -> (→"Acceleration (m/s^2)":dbl)
    n368 = global read "podGlobals_9066.vi" "Velocity (m/s)"() -> (→"Velocity (m/s)":dbl)
    n369 = global read "podGlobals_9066.vi" "Battery Pressure (atm)"() -> (→"Battery Pressure (atm)":dbl)
    n370 = global read "podGlobals_9066.vi" "Battery Temperature (C)"() -> (→"Battery Temperature (F)":dbl)
    n371 = global read "podGlobals_9066.vi" "Internal Pressure (atm)"() -> (→"Internal Pressure (atm)":dbl)
    n372 = global read "podGlobals_9066.vi" "Internal Temperature (C)"() -> (→"Internal Temperature (F)":dbl)
    n373 = global read "podGlobals_9066.vi" "Progress"() -> (→"Progress":dbl)
    n374 = global read "podGlobals_9066.vi" "Battery Voltage"() -> (→"Battery Voltage":dbl)
    n375 = global read "podGlobals_9066.vi" "Front Brake Engaged"() -> (→"Front Brake Engaged":bool)
    n376 = global read "podGlobals_9066.vi" "Flight Time (s)"() -> (→"Flight Time (s)":dbl)
    n377 = global read "podGlobals_9066.vi" "On Time (s)"() -> (→"On Time (s)":dbl)
    n378 = global read "podGlobals_9066.vi" "Coast Time (s)"() -> (→"Coast Time (s)":dbl)
    n379 = global read "podGlobals_9066.vi" "Start Time (s)"() -> (→"Start Time (s)":dbl)
    n380 = global read "podGlobals_9066.vi" "Pusher Engaged"() -> (→"Pusher Engaged":bool)
    n381 = global read "podGlobals_9066.vi" "BatTemp"() -> (→"Battery Temperature":bool)
    n382 = global read "podGlobals_9066.vi" "BatPress"() -> (→"Battery Pressure":bool)
    n383 = global read "podGlobals_9066.vi" "BatVolt"() -> (→"Battery Voltage":bool)
    n384 = global read "podGlobals_9066.vi" "READY"() -> (→"READY":bool)
    n385 = global read "podGlobals_9066.vi" "Back Brake Engaged"() -> (→"Back Brake Engaged":bool)
    n386 = global read "podGlobals_9066.vi" "Z-Height FR (mm)"() -> (→"FR:":dbl)
    n387 = global read "podGlobals_9066.vi" "Z-Height BR (mm)"() -> (→"BR:":dbl)
    n388 = global read "podGlobals_9066.vi" "Z-Height FL (mm)"() -> (→"FL:":dbl)
    n389 = global read "podGlobals_9066.vi" "Z-Height BL (mm)"() -> (→"BL:":dbl)
    n390 = global read "podGlobals_9066.vi" "IntTemp"() -> (→"Internal Temperature":bool)
    n391 = global read "podGlobals_9066.vi" "Accel"() -> (→"Acceleration":bool)
    n392 = global read "podGlobals_9066.vi" "Vel"() -> (→"Velocity":bool)
    n393 = global read "podGlobals_9066.vi" "IntPress"() -> (→"Internal Pressure":bool)
    n394 = global read "podGlobals_9066.vi" "Latched"() -> (→"Latched":bool)
    n395 = node-c288() -> ()  [unwired: 1 in, 1 out]
  }
  n396 = node-c288(w13) -> ()  [unwired: 1 out]
  n397 = node-c288(w6) -> ()  [unwired: 1 out]
